vi "Delete empty header content.vi"(8 "error in (no error)":errorcluster, 11 "Save Image in":refnum<class "Save Image.lvclass">) -> (0 "error out":errorcluster, 3 "Save Image out":refnum<class "Save Image.lvclass">)   [LabVIEW 2018, in "Save Image.lvclass"]
uses:
  Save Image.lvclass
  Save Image.lvclass/Save Image.ctl
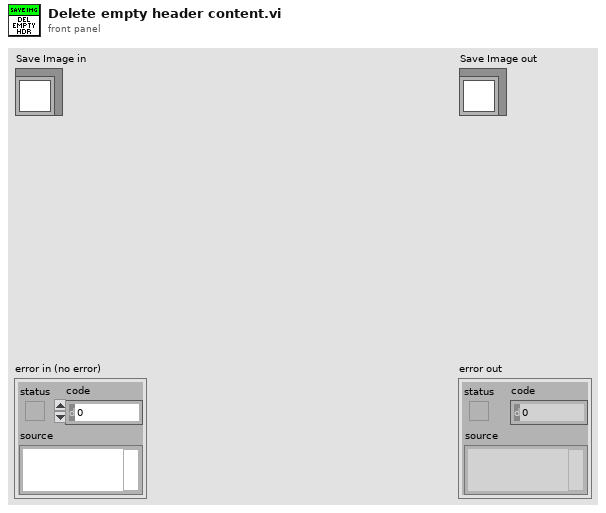
[diagram p1: front panel]
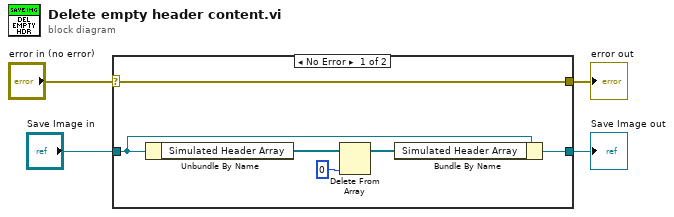
[diagram p0: block diagram]
diagram:
  n1 = case shown="No Error" "error in (no error)" {
    selector: "error in (no error)" -> [w5 w12]
    tunnel: [w5 w12] -> w3
    tunnel: [w10 w11] -> w1
    tunnel: "Save Image in" -> [w6 w11]
    frame No Error {
      n2 = Unbundle By Name(w6) -> ("Simulated Header Array"=w9:refnum<class "Simulated_Header.lvclass">[])
      n3 = Delete From Array(array=w9, index=0) -> (array with subset deleted=w7:refnum<class "Simulated_Header.lvclass">[])  [unwired: 1 in, 1 out]
      n4 = Bundle By Name(cluster=w6, "Simulated Header Array"=w7) -> (w10:refnum<class "Save Image.lvclass">)
    }
    frame Error {
    }
  }
  "error out" <- w3
  "Save Image out" <- w1
